vi "RH_FGEN_Close.vi"(8 "error in":errorcluster, 10 "Reset":bool, 11 "FGEN Session In":refnum<k15>) -> (0 "error out":errorcluster)   [LabVIEW 2023, in "ResourceHandling.lvlib"]
doc: "Close the session and eventually resets it"
uses:
  ResourceHandling.lvlib
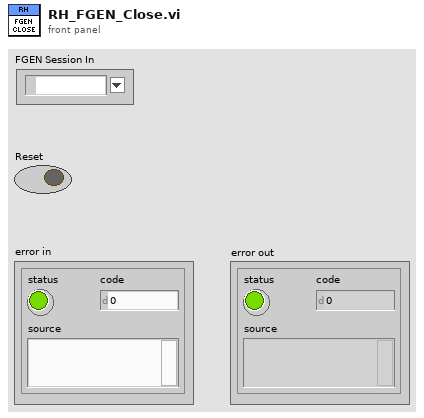
[diagram p1: front panel]
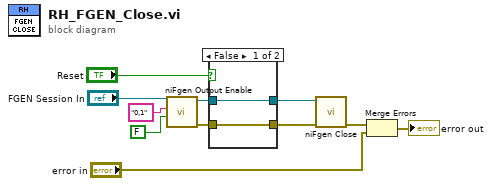
[diagram p0: block diagram]
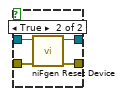
[diagram p2: hidden frame]
diagram:
  n1 = call <instrlib>:"niFgen Output Enable.vi"("Output Enable (default: True)"=FALSE, "Channel Name"="0,1", "Instrument Handle"="FGEN Session In") -> ("error out"=w3:errorcluster, "Instrument Handle Out"=w6:refnum<k15>)  [unwired: 7 in]
  n2 = case shown="False" "Reset" {
    tunnel: [w12 w17] -> w4
    tunnel: [w13 w16] -> w5
    tunnel: w6 -> [w13 w15]
    tunnel: w3 -> [w12 w14]
    frame False {
    }
    frame True {
      n3 = call <instrlib>:"niFgen Reset Device.vi"("error in (no error)"=w14, "Instrument Handle"=w15) -> ("error out"=w17:errorcluster, "Instrument Handle Out"=w16:refnum<k15>)  [unwired: 8 in]
    }
  }
  n4 = call <instrlib>:"niFgen Close.vi"("error in (no error)"=w4, "Instrument Handle"=w5) -> ("error out"=w10:errorcluster)  [unwired: 9 in]
  n5 = Merge Errors(w10, "error in") -> (→"error out":errorcluster)
